vi "HP34401_close.vi"(8 "error in":errorcluster, 11 "VISA in":refnum<visa-resource-name>) -> (0 "error out":errorcluster)   [LabVIEW 2020]
uses:
  <vilib>/Instr/_visa.llb/VISA GPIB Control REN Mode.ctl
  drivers/HP34401A/Agilent 34401.lvlib
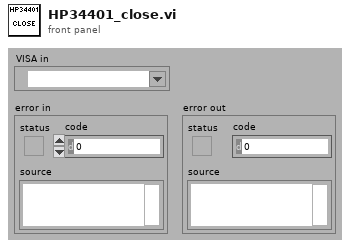
[diagram p1: front panel]
types:
  T1 = typedef "VISA GPIB Control REN Mode.ctl" = u16
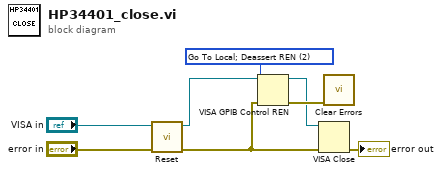
[diagram p0: block diagram]
diagram:
  w6 = T1 2 items=["Deassert REN", "Assert REN", "Go To Local; Deassert REN ", "Assert REN; Address Device", "Local Lockout (Addressed Devices)", "Local Lockout (This Device)", "Go To Local"] ("Mode")
  n1 = call "Reset.vi"("error in (no error)"="error in", "VISA resource name"="VISA in") -> ("error out"=w3:errorcluster, "VISA resource name out"=w1:refnum<visa-resource-name>)  [unwired: 8 in]
  n2 = VISA GPIB Control REN(8:w3, 10:w6, 11:w1) -> (0:w8:errorcluster, 3:w7:refnum<visa-resource-name>)
  n3 = VISA Close(VISA resource name=w7, error in (no error)=w3) -> (error out=→"error out":errorcluster)
  n4 = call <vilib>:"Clear Errors.vi"("error in (no error)"=w8) -> ()  [unwired: 5 in, 2 out]
